vi "Read Data.vi"(2 "Selected data":dbl[][](array[numeric])) -> (5 "# OK":i32, 6 "# Over Range":i32, 7 "Data Point":dbl, 8 "# Missing Pulses":i32, 9 "# Saturated":i32)   [LabVIEW 2009]
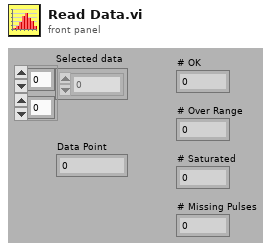
[diagram p1: front panel]
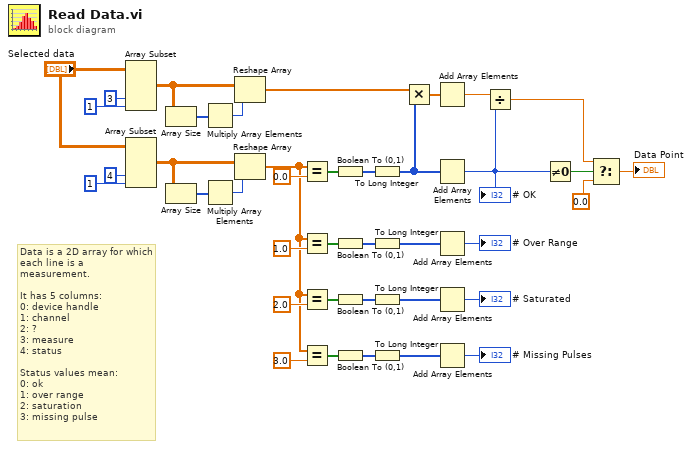
[diagram p0: block diagram]
diagram:
  # "Data is a 2D array for which\neach line is a measurement.\n\nIt has 5 columns:\n0: device handle\n1: channel\n2: ?\n3: measure\n4: status\n\nStatus values mean:\n0: ok\n1: over range\n2: saturation\n3: missing pulse"
  n1 = Array Subset(array="Selected data", index (col)=3 ("index"), length (col)=1 ("length")) -> (w36:dbl[][])  [unwired: 2 in]
  n2 = Array Subset(array="Selected data", index (col)=4 ("index"), length (col)=1 ("length")) -> (w33:dbl[][])  [unwired: 2 in]
  n3 = Array Size(array=w36) -> (size(s)=w37:i32[])
  n4 = Array Size(array=w33) -> (size(s)=w32:i32[])
  n5 = Multiply Array Elements(1:w37) -> (0:w35:i32)
  n6 = Multiply Array Elements(1:w32) -> (0:w34:i32)
  n7 = Reshape Array(w36, w35) -> (w22:dbl[])
  n8 = Reshape Array(w33, w34) -> (w24:dbl[])
  n9 = Equal?(x=w24, y=0.0) -> (x = y?=w23:bool[])
  n10 = Equal?(x=w24, y=1.0) -> (x = y?=w11:bool[])
  n11 = Equal?(x=w24, y=2.0) -> (x = y?=w10:bool[])
  n12 = Equal?(x=w24, y=3.0) -> (x = y?=w9:bool[])
  n13 = Boolean To (0,1)(Boolean=w23) -> (0, 1=w21:i16[])
  n14 = Boolean To (0,1)(Boolean=w11) -> (0, 1=w14:i16[])
  n15 = Boolean To (0,1)(Boolean=w10) -> (0, 1=w13:i16[])
  n16 = Boolean To (0,1)(Boolean=w9) -> (0, 1=w12:i16[])
  n17 = To Long Integer(number=w21) -> (32bit integer=w20:i32[])
  n18 = To Long Integer(number=w14) -> (32bit integer=w8:i32[])
  n19 = To Long Integer(number=w13) -> (32bit integer=w7:i32[])
  n20 = To Long Integer(number=w12) -> (32bit integer=w6:i32[])
  n21 = Multiply(x=w22, y=w20) -> (x*y=w19:dbl[])
  n22 = Add Array Elements(numeric array=w19) -> (sum=w18:dbl)
  n23 = Add Array Elements(numeric array=w20) -> (sum=w5:i32)
  "# OK" <- w5
  n24 = Add Array Elements(numeric array=w8) -> (sum=→"# Over Range":i32)
  n25 = Add Array Elements(numeric array=w7) -> (sum=→"# Saturated":i32)
  n26 = Add Array Elements(numeric array=w6) -> (sum=→"# Missing Pulses":i32)
  n27 = Divide(x=w18, y=w5) -> (x/y=w16:dbl)
  n28 = Not Equal To 0?(x=w5) -> (x != 0?=w17:bool)
  n29 = Select(t=w16, s=w17, f=0.0) -> (s? t:f=→"Data Point":dbl)
